vi "Vector Norm.vi"(11 "Vector":cluster{"X":sgl, "Y":sgl, "Z":sgl}) -> (3 "Norm":sgl)   [LabVIEW 2020, in "3D Plot.lvclass"]
uses:
  <vilib>/Math Plots/3D Math Plots/3D Plot/3D Plot/3D Plot.lvclass
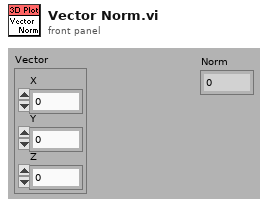
[diagram p1: front panel]
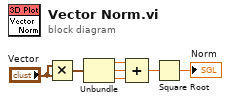
[diagram p0: block diagram]
diagram:
  n1 = Multiply(x="Vector", y="Vector") -> (x*y=w7:cluster{"X":sgl, "Y":sgl, "Z":sgl})
  n2 = Unbundle(w7) -> ("X"=w6:sgl, "Y"=w5:sgl, "Z"=w4:sgl)
  n3 = Compound Arithmetic op=ADD(w6, w5, w4) -> (w3:sgl)
  n4 = Square Root(x=w3) -> (sqrt(x)=→"Norm":sgl)
